vi "SQL Select.vi"(11 "variant":variant) -> (3 "SQL":string caption="SQL with colums inserted before FROM")   [LabVIEW 2021]
doc: "Formats an array of column names before the \"FROM\" keyword in the input SQL INSERT statement. For use when working with a variable list of columns."
uses:
  <vilib>/JDP Science/JDP Science Common Utilities/JDP Utility.lvlib
  <vilib>/Utility/Data Type/NI_Data Type.lvlib
panel:
  out "name":string
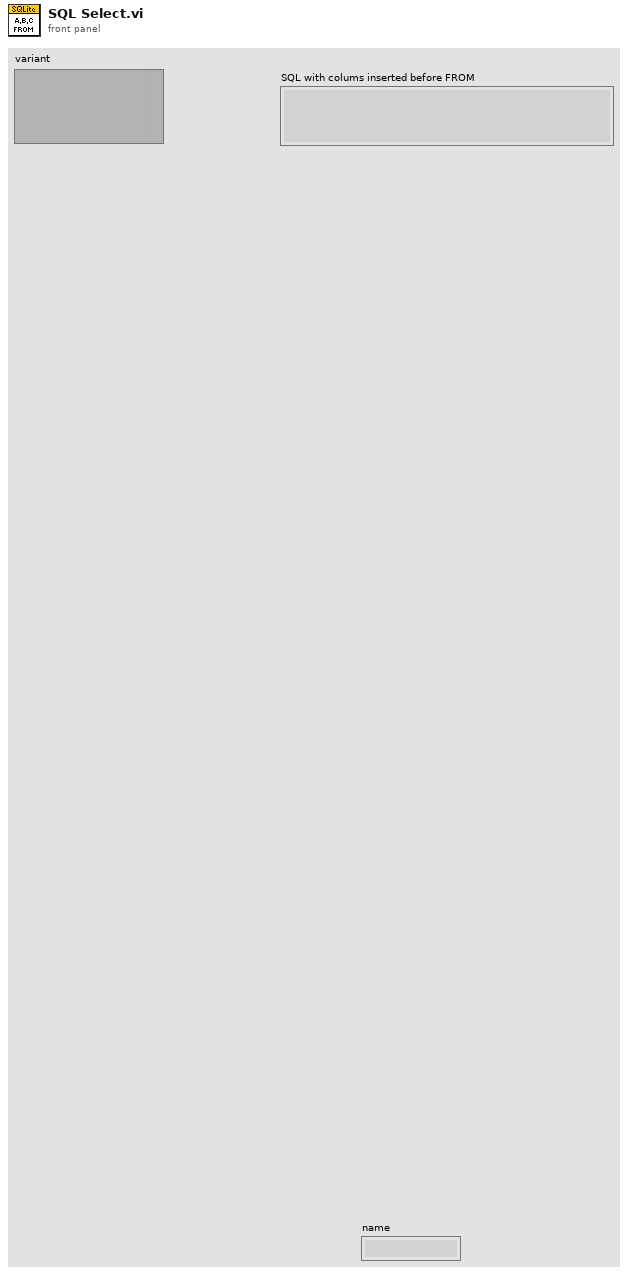
[diagram p1: front panel]
types:
  T1 = typedef "NI_Data Type.lvlib/Data Type.ctl" = enum8{"Invalid Type", "Void", "I8", "I16", "I32", "I64", "U8", "U16", "U32", "U64", "Single Float", "Double Float", "Extended Float", "Single Complex", "Double Complex", "Extended Complex", "Enum U8", "Enum U16", "Enum U32", "Enum U64", "Single Float With Unit", "Double Float With Unit", "Extended Float With Unit", "Single Complex with Unit", "Double Complex with Unit", "Extended Complex with Unit", "Boolean", "String", "Path", "Picture", "Tag", "Array", "Cluster", "Variant", "LV Variant", "Waveform", "Timestamp", "Digital Waveform", "Digital Data", "ExpressData", "Refnum", "External Data", "VI", "Poly VI", "LabVIEW Class Instance", "Fixed Point", "Set Collection", "Map Collection"}
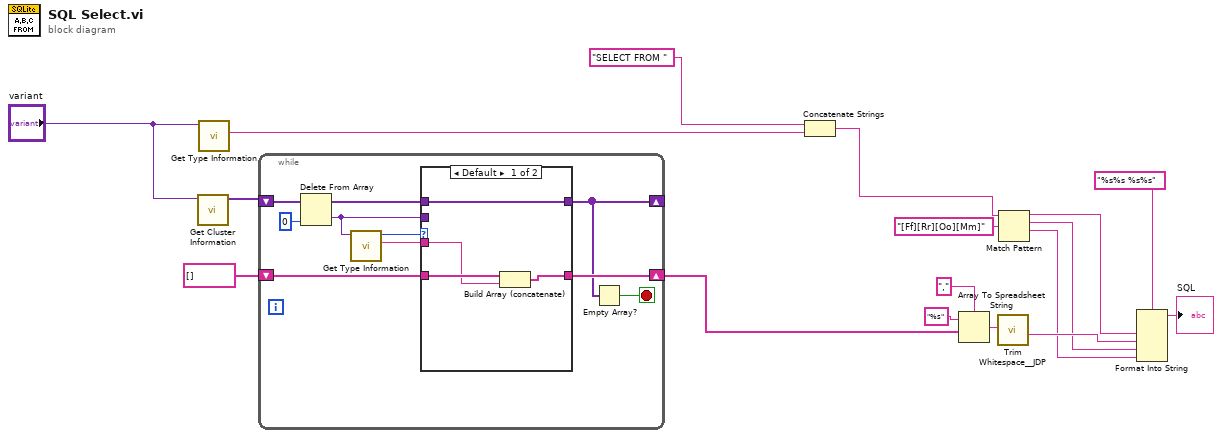
[diagram p0: block diagram]
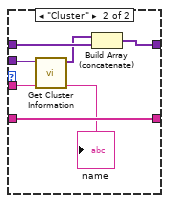
[diagram p2: hidden frame]
diagram:
  n1 = call <vilib>:"Get Cluster Information.vi"("variant"="variant") -> ("cluster elements"=w6:variant[])  [unwired: 9 in, 1 out]
  n2 = call <vilib>:"Get Type Information.vi"("variant"="variant") -> ("name"=w3:string)  [unwired: 6 in, 4 out]
  n3 = while {
    shift-right: [w18] -> _
    shift-left: w6 -> [w27]
    shift-right: [w22] -> w1
    shift-left: string[] [] -> [w23]
    stop <- w25 stop-if-true
    n4 = Delete From Array(array=w27, index=0) -> (deleted portion=w19:variant, array with subset deleted=w24:variant[])  [unwired: 1 in]
    n5 = call <vilib>:"Get Type Information.vi"("variant"=w19) -> ("name"=w20:string, "type"=w21:T1)  [unwired: 6 in, 3 out]
    n6 = case shown="Default" w21 {
      tunnel: w24 -> [w31 w37]
      tunnel: w19 -> [_ w34]
      tunnel: [w31 w36] -> w18
      tunnel: w23 -> [w30 w35]
      tunnel: [w28 w35] -> w22
      tunnel: w20 -> [w29 w32]
      frame Default {
        n7 = Build Array (concatenate)(w30, w29) -> (w28:string[])
      }
      frame "Cluster" {
        n8 = call <vilib>:"Get Cluster Information.vi"("variant"=w34) -> ("cluster elements"=w33:variant[])  [unwired: 9 in, 1 out]
        n9 = Build Array (concatenate)(w33, w37) -> (w36:variant[])
        "name" <- w32
      }
    }
    n10 = Empty Array?(array=w18) -> (empty?=w25:bool)
  }
  n11 = Concatenate Strings("SELECT FROM " ("SQL containing FROM clause"), w3) -> (w2:string)
  n12 = Array To Spreadsheet String(delimiter (Tab)=",", array=w1, 3:"%s" ("format string")) -> (spreadsheet string=w15:string)
  n13 = call <vilib>:"Trim Whitespace__JDP.vi"("String in"=w15) -> ("String out"=w10:string)  [unwired: 6 in]
  n14 = Match Pattern(string=w2, regular expression="[Ff][Rr][Oo][Mm]") -> (before substring=w11:string, match substring=w9:string, after substring=w8:string)  [unwired: 1 in, 1 out]
  n15 = Format Into String(format string="%s%s %s%s", w11, w10, w9, w8) -> (resulting string=→"SQL":string)  [unwired: 2 in, 1 out]
